vi "Register for Events.vi"(8 "error in (no error)":errorcluster, 11 "Slave Test Runner In":refnum<class "Slave Test Runner.lvclass">) -> (0 "error out":errorcluster, 2 "Event Registration Refnum":refnum<event-registration>, 3 "Slave Test Runner Out":refnum<class "Slave Test Runner.lvclass">)   [LabVIEW 2020, in "Slave Test Runner.lvclass"]
uses:
  Slave Test Runner.lvclass
  Test Case/LUnit Test Case.lvclass
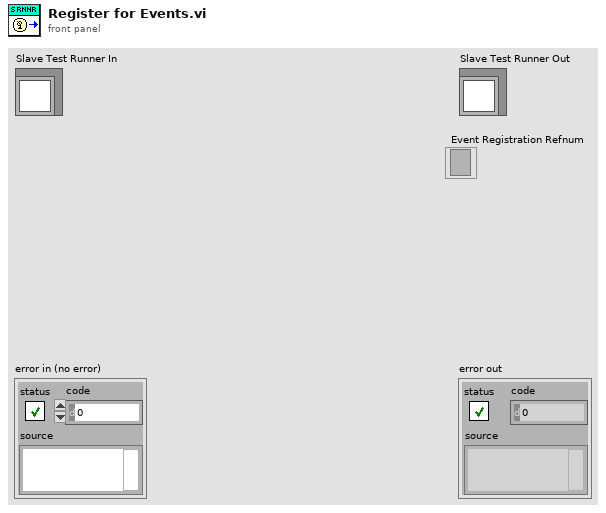
[diagram p1: front panel]
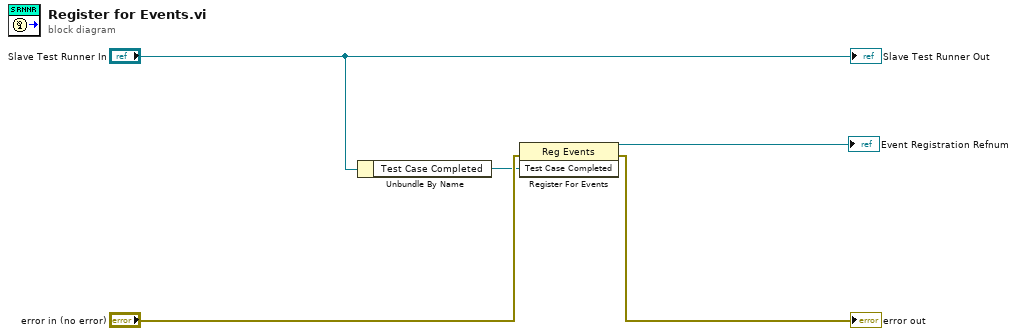
[diagram p0: block diagram]
diagram:
  n1 = Unbundle By Name("Slave Test Runner In") -> ("Test Case Completed"=w2:refnum<user-event>)
  n2 = register-events(error in="error in (no error)", w2) -> (reference out=→"Event Registration Refnum":refnum<event-registration>, error out=→"error out":errorcluster)  [unwired: 1 in]
  "Slave Test Runner Out" <- "Slave Test Runner In"
